vi "DeviceRead.vi"(4 "error in (no error)":errorcluster, 6 "DeviceKey In":string, 7 "USBLib In":refnum<k24>) -> (0 "error out":errorcluster, 1 "Response":string, 2 "DeviceKey Out":string, 3 "USBLib Out":refnum<k24>)   [LabVIEW 2009]
uses:
  C:/Samples/LabVIEW/UseDeviceKey/LabVIEW 2009/UseDeviceKey (with Device VIs)/UsbDllWrap.dll
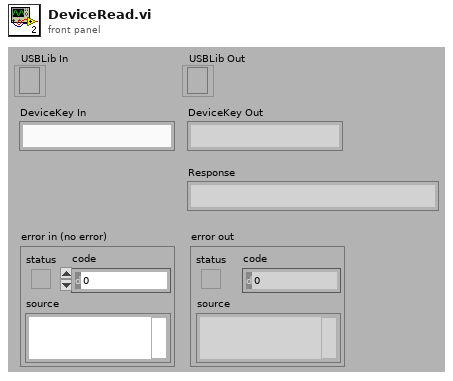
[diagram p1: front panel]
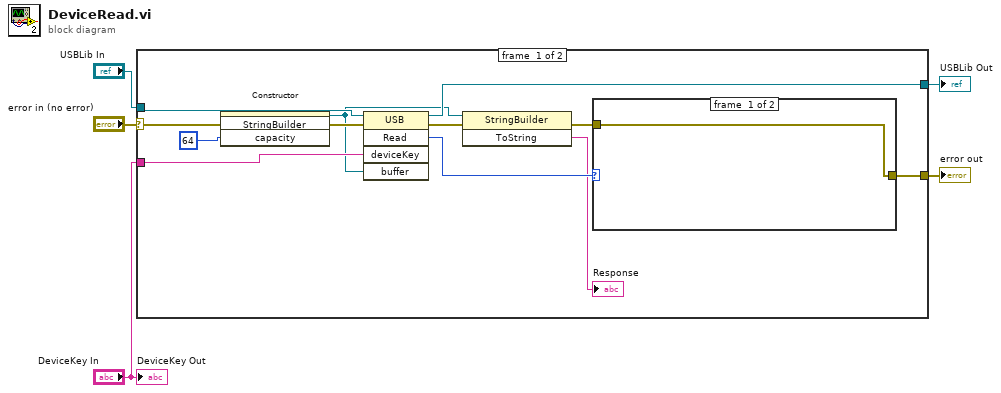
[diagram p0: block diagram]
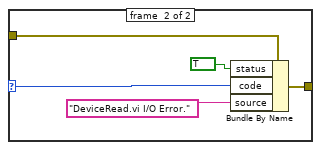
[diagram p2: hidden frame]
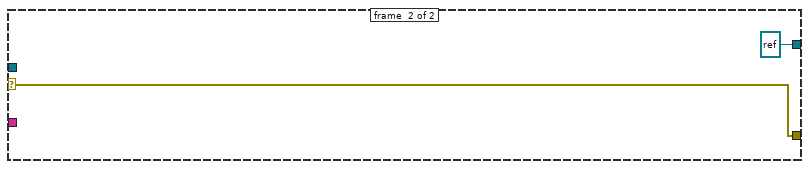
[diagram p3: hidden frame]
diagram:
  n1 = case shown="No Error" "error in (no error)" {
    selector: "error in (no error)" -> [w13 w25]
    tunnel: [w8 w25] -> w4
    tunnel: "DeviceKey In" -> [w17 _]
    tunnel: "USBLib In" -> [w16 _]
    tunnel: [w15 refnum<k24> refnum ("USBLib In")] -> w1
    frame #0 {
      n2 = constructor class="StringBuilder"(error in=w13, "capacity"=64) -> (reference out=w6:refnum<k24>, error out=w12:errorcluster)  [unwired: 2 in, 2 out]
      n3 = invoke class="USB" method="Read"(reference=w16, error in=w12, "deviceKey"=w17, "buffer"=w6) -> (reference out=w15:refnum<k24>, error out=w11:errorcluster, "Read"=w10:i32)  [unwired: 1 in, 2 out]
      n4 = invoke class="StringBuilder" method="ToString"(reference=w6, error in=w11) -> (error out=w9:errorcluster, "ToString"=→"Response":string)  [unwired: 1 in, 1 out]
      n5 = case shown="1, Default" w10 {
        selector: w10 -> [_ w19]
        tunnel: w9 -> [w18 w21]
        tunnel: [w18 w20] -> w8
        frame #0 {
        }
        frame #1 {
          n6 = Bundle By Name(cluster=w21, "status"=TRUE, "code"=w19, "source"="DeviceRead.vi I/O Error.") -> (w20:errorcluster)
        }
      }
    }
    frame #1 {
    }
  }
  "error out" <- w4
  "USBLib Out" <- w1
  "DeviceKey Out" <- "DeviceKey In"
